vi "Loop_ACT_Claw_Rotation.vi"() -> ()   [LabVIEW 2017, in "Lift.lvlib"]
uses:
  Lift.lvlib
  _SHARE ALL/TypeDef Share All/CLUSTER_TalonInput.ctl
  System Drivers/Phoenix-LabVIEW/Motor Controller/Controls/CTRE_Phoenix_MotorControl_ControlMode.ctl
  _SHARE ALL/RoboRio Share All/SRX Share All/TypeDefs SRX/Cluster_SRX_PIDF.ctl
  _SHARE ALL/TypeDef Share All/CONTROL_PositonGraph.ctl
  CLUSTER_ACT_Lift Output.ctl
  _SHARE ALL/RoboRio Share All/SRX Share All/TypeDefs SRX/Cluster_SRX_General Data.ctl
  _SHARE ALL/RoboRio Share All/SRX Share All/TypeDefs SRX/Cluster_SRX_Common Runtime Data.ctl
  _SHARE ALL/RoboRio Share All/SRX Share All/TypeDefs SRX/Cluster_SRX_Error Calculations.ctl
  _SHARE ALL/RoboRio Share All/SRX Share All/TypeDefs SRX/Cluster_SRX_Voltage Out Data.ctl
  _SHARE ALL/RoboRio Share All/SRX Share All/TypeDefs SRX/Cluster_SRX_Sensor Out Data.ctl
  _SHARE ALL/RoboRio Share All/SRX Share All/TypeDefs SRX/Cluster_SRX_Sensor Quad Data.ctl
  _SHARE ALL/RoboRio Share All/SRX Share All/TypeDefs SRX/Cluster_SRX_Analog In Data.ctl
  _SHARE ALL/RoboRio Share All/SRX Share All/TypeDefs SRX/Cluster_SRX_PWM Sensor Data.ctl
  _SHARE ALL/RoboRio Share All/SRX Share All/TypeDefs SRX/Cluster_SRX_F and R Limit Indicators.ctl
  TypeDef/CLUSTER_PID.ctl
  Globals/Global_Device_IDs.vi
  _SHARE ALL/Global Share All/Global_STOP.vi
  Global_SM Write_Data Out.vi
  Global_ACT Write_Data Out.vi
panel:
  out "Rotation Output":T1 {"Common Runtime Data Out"."Temp" format="%.1f"; "Common Runtime Data Out"."Voltage"."Bus" format="%.3f"; "Common Runtime Data Out"."Voltage"."Output" format="%.3f"; "Common Runtime Data Out"."Voltage"."Percent" format="%.3f"; "Common Runtime Data Out"."Current" format="%.2f"}
  in  "Display Graph":bool
  out "Position Closed Loop Plots":T11
  out "Rotation Input":T12 {"Talon Mode" items=["PercentOutput"=0, "Position"=1, "Velocity"=2, "Current"=3, "Follower"=5, "MotionProfile"=6, "MotionMagic"=7, "MotionMagicArc"=8, "MotionProfileArc"=10, "Disabled"=15]}
  out "Cycle Time (S)":dbl format="%.3g"
  in  "Target Time(ms)":u32=50
  # "C"
  # "Units"
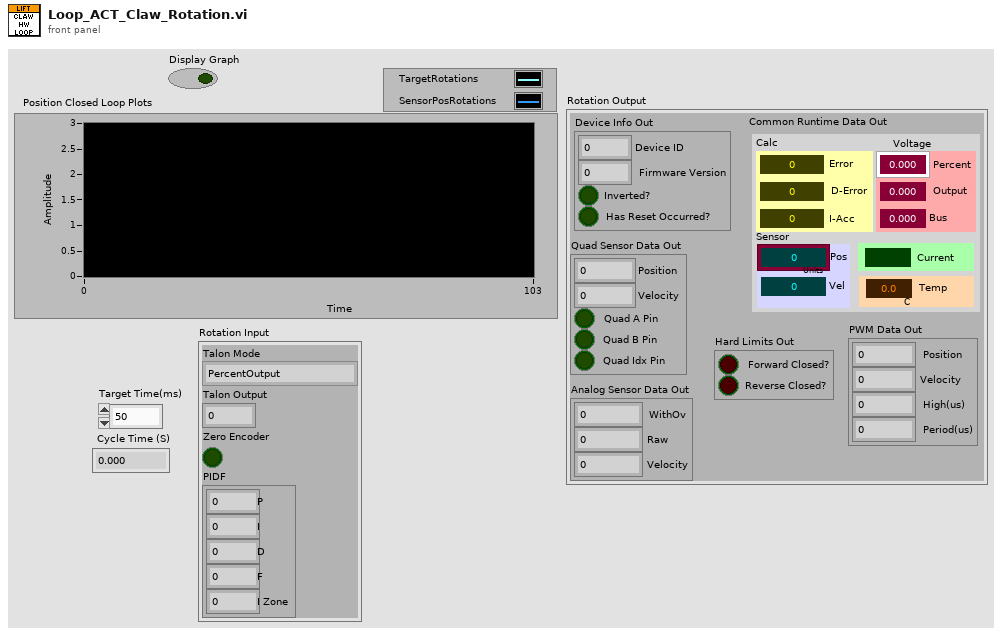
[diagram p1: front panel]
types:
  T1 = typedef "Lift.lvlib/CLUSTER_ACT_Lift Output.ctl" = cluster{"Device Info Out":T2, "Common Runtime Data Out":T3, "Quad Sensor Data Out":T7, "Analog Sensor Data Out":T8, "PWM Data Out":T9, "Hard Limits Out":T10}
  T2 = typedef "Cluster_SRX_General Data.ctl" = cluster{"Device ID":i32, "Firmware Version":i32, "Inverted?":bool, "Has Reset Occurred?":bool}
  T3 = typedef "Cluster_SRX_Common Runtime Data.ctl" = cluster{"Calc":T4, "Voltage ":T5, "Sensor":T6, "Current":dbl, "Temp":dbl}
  T4 = typedef "Cluster_SRX_Error Calculations.ctl" = cluster{"Error":i32, "D-Error":dbl, "I-Acc":dbl}
  T5 = typedef "Cluster_SRX_Voltage Out Data.ctl" = cluster{"Percent":dbl, "Output":dbl, "Bus":dbl}
  T6 = typedef "Cluster_SRX_Sensor Out Data.ctl" = cluster{"Pos":i32, "Vel":i32}
  T7 = typedef "Cluster_SRX_Sensor Quad Data.ctl" = cluster{"Position":i32, "Velocity":i32, "Quad A Pin":bool, "Quad B Pin":bool, "Quad Idx Pin":bool}
  T8 = typedef "Cluster_SRX_Analog In Data.ctl" = cluster{"WithOv":i32, "Raw":i32, "Velocity":i32}
  T9 = typedef "Cluster_SRX_PWM Sensor Data.ctl" = cluster{"Position":i32, "Velocity":i32, "High(us)":i32, "Period(us)":i32}
  T10 = typedef "Cluster_SRX_F and R Limit Indicators.ctl" = cluster{"Forward Closed?":bool, "Reverse Closed?":bool}
  T11 = typedef "CONTROL_PositonGraph.ctl" = cluster{dbl, "Position (Raw Sensor Units)":i32}
  T12 = typedef "CLUSTER_TalonInput.ctl" = cluster{"Talon Mode":T13, "Talon Output":dbl, "Zero Encoder":bool, "PIDF":T14}
  T13 = typedef "CTRE_Phoenix_MotorControl_ControlMode.ctl" = u16
  T14 = typedef "Cluster_SRX_PIDF.ctl" = cluster{"P":dbl, "I":dbl, "D":dbl, "F":dbl, "I Zone":dbl}
  T15 = typedef "CLUSTER_PID.ctl" = cluster{"P":dbl, "I":dbl, "D":dbl, "F":dbl, "I Zone":dbl}
  T16 = typedef "CLUSTER_Arm_Device_IDs.ctl" = cluster{"Rotation Setup":T17, "Telescope Setup":T17, "Rotation Slave Setup":T17, "Telescope Slave Setup":T17, "Claw Rotation Setup":T17}
  T17 = typedef "CLUSTER_Talon_Setup.ctl" = cluster{"Talon SRX ID":u8, "PhaseSensor":bool, "Invert Motor?":bool, "Phoenix Feedback Select":T18, "pidLoopldx":i32, "PID":T15}
  T18 = typedef "CTRE_Phoenix_MotorControl_FeedbackDevice.ctl" = i8
  T19 = typedef "WPI_MotorControlDeviceRef.ctl" = cluster{"DeviceStatus":errorcluster, "Type":T20, "PWM":cluster{"PWM Channel":T21, "DeadBand":T22}, "CAN":cluster{"Device Number":u8, "SetOutput VI Ref":variant, "GetOutput VI Ref":variant, "Enable VI Ref":variant, "Disable VI Ref":variant, "Data":variant}, "Invert":bool, "DIO PWM":cluster{"PWM \"Enable\" Channel":T21, "DIOChannel":T23, "PWM Rate":dbl}}
  T20 = typedef "WPI_MotorControlType.ctl" = enum16{"PWM", "CAN", "DIO PWM"}
  T21 = typedef "FPGA_DIOPWMChannel.ctl" = enum8{"PWM 0", "PWM 1", "PWM 2", "PWM 3", "PWM 4", "PWM 5", "PWM 6", "PWM 7", "PWM 8", "PWM 9", "PWM MXP 0", "PWM MXP 1", "PWM MXP 2", "PWM MXP 3", "PWM MXP 4", "PWM MXP 5", "PWM MXP 6", "PWM MXP 7", "PWM MXP 8", "PWM MXP 9", "Invalid"}
  T22 = typedef "WPI_PWMDeadband.ctl" = cluster{"Name":string, "maxPositivePwm":i32, "minPositivePwm":i32, "centerPwm":i32, "maxNegativePwm":i32, "minNegativePwm":i32, "angularRange":u16}
  T23 = typedef "FPGA_DIOChannel.ctl" = enum8{"DIO 0", "DIO 1", "DIO 2", "DIO 3", "DIO 4", "DIO 5", "DIO 6", "DIO 7", "DIO 8", "DIO 9", "DIO MXP 0", "DIO MXP 1", "DIO MXP 2", "DIO MXP 3", "DIO MXP 4", "DIO MXP 5", "DIO MXP 6", "DIO MXP 7", "DIO MXP 8", "DIO MXP 9", "DIO MXP 10", "DIO MXP 11", "DIO MXP 12", "DIO MXP 13", "DIO MXP 14", "DIO MXP 15", "SPI Port CS1", "SPI Port CS2", "SPI Port CS3", "SPI Port MISO", "SPI Port MOSI", "Invalid"}
  T24 = cluster{"PhoenixMotorControlDevRef":T19, "Claw Rotation Output":T1, "Claw Rotation Input":T12, "Target Time(ms)":u32, "Current Time":timestamp, "Previous Time":timestamp, "Cycle Time (S)":dbl, "Last PID":T15}
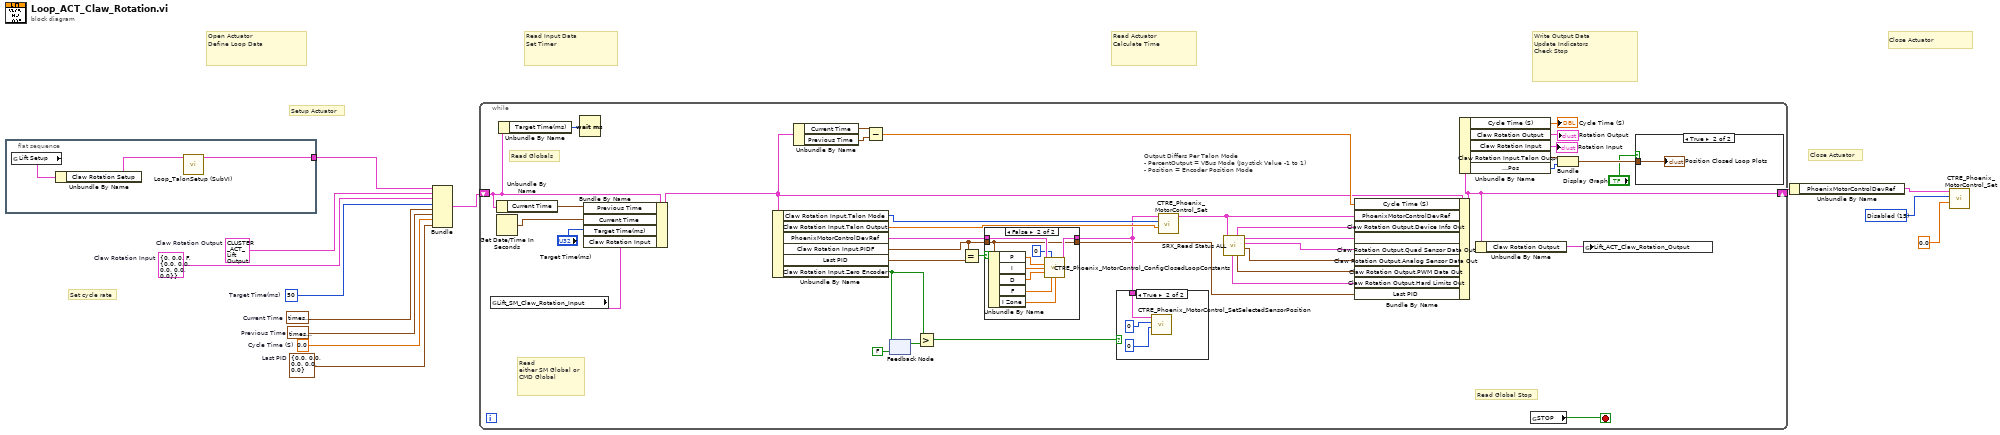
[diagram p0: block diagram]
diagram:
  w1 = T1 {"Device Info Out"={"Device ID"=0, "Firmware Version"=0, "Inverted?"=FALSE, "Has Reset Occurred?"=FALSE}, "Common Runtime Data Out"={"Calc"={"Error"=0, "D-Error"=0.0, "I-Acc"=0.0}, "Voltage "={"Percent"=0.0, "Output"=0.0, "Bus"=0.0}, "Sensor"={"Pos"=0, "Vel"=0}, "Current"=0.0, "Temp"=0.0}, "Quad Sensor Data Out"={"Position"=0, "Velocity"=0, "Quad A Pin"=FALSE, "Quad B Pin"=FALSE, "Quad Idx Pin"=FALSE}, "Analog Sensor Data Out"={"WithOv"=0, "Raw"=0, "Velocity"=0}, "PWM Data Out"={"Position"=0, "Velocity"=0, "High(us)"=0, "Period(us)"=0}, "Hard Limits Out"={"Forward Closed?"=FALSE, "Reverse Closed?"=FALSE}}  # Claw Rotation Output
  w3 = T15 {"P"=0.0, "I"=0.0, "D"=0.0, "F"=0.0, "I Zone"=0.0}  # Last PID
  w5 = T13 15 items=["PercentOutput"=0, "Position"=1, "Velocity"=2, "Current"=3, "Follower"=5, "MotionProfile"=6, "MotionMagic"=7, "MotionMagicArc"=8, "MotionProfileArc"=10, "Disabled"=15] ("Control Mode")
  w7 = T12 {"Talon Mode"=0, "Talon Output"=0.0, "Zero Encoder"=FALSE, "PIDF"={"P"=0.0, "I"=0.0, "D"=0.0, "F"=0.0, "I Zone"=0.0}}  # Claw Rotation Input
  w8 = 0.0  # Cycle Time (S)
  w13 = timestamp(0 s since 1904-01-01)  # Previous Time
  w12 = timestamp(0 s since 1904-01-01)  # Current Time
  w11 = u32 50  # Target Time(ms)
  # "Close Actuator"
  # "Write Output Data\nUpdate Indicators\nCheck Stop"
  # "Read Actuator\nCalculate Time"
  # "Read Input Data\nSet Timer"
  # "Open Actuator\nDefine Loop Data"
  # "Set cycle rate"
  # "Close Actuator"
  # "Setup Actuator"
  n1 = flat-sequence {
    tunnel: [w14] -> w2
    frame #0 {
      n2 = global read "Global_Device_IDs.vi" "Lift Setup"() -> (w16:T16)
      n3 = Unbundle By Name(w16) -> ("Claw Rotation Setup"=w15:T17)
      n4 = call "Loop_TalonSetup (SubVI).vi"("Talon Setup"=w15) -> ("PhoenixMotorControlDevRef"=w14:T19)  [unwired: 10 in]
    }
  }
  n5 = Bundle("PhoenixMotorControlDevRef"=w2, "Claw Rotation Output"=w1, "Claw Rotation Input"=w7, "Target Time(ms)"=w11, "Current Time"=w12, "Previous Time"=w13, "Cycle Time (S)"=w8, "Last PID"=w3) -> (w10:T24)  [unwired: 1 in]
  n6 = while {
    shift-right: [w47] -> w9
    shift-left: w10 -> [w49]
    stop <- w55 stop-if-true
    # "Output Differs Per Talon Mode\n- PercentOutput = VBus Mode (Joystick Value -1 to 1)\n- Position = Encoder Position Mode"
    # "Read\neither SM Global or CMD Global"
    # "Read Globals"
    # "Read Global Stop"
    n7 = global read "Global_SM Write_Data Out.vi" "Lift_SM_Claw_Rotation_Input"() -> (w43:T12)
    n8 = Unbundle By Name(w49) -> ("Current Time"=w53:timestamp)
    n9 = Get Date/Time In Seconds() -> (seconds since 1Jan1904=w54:timestamp)
    n10 = Unbundle By Name(w49) -> ("Target Time(ms)"=w48:u32)
    n11 = Wait (ms)(milliseconds to wait=w48) -> ()  [unwired: 1 out]
    n12 = Bundle By Name(cluster=w49, "Previous Time"=w53, "Current Time"=w54, "Target Time(ms)"="Target Time(ms)", "Claw Rotation Input"=w43) -> (w36:T24)
    n13 = Unbundle By Name(w36) -> ("Claw Rotation Input.Talon Mode"=w42:T13, "Claw Rotation Input.Talon Output"=w41:dbl, "PhoenixMotorControlDevRef"=w35:T19, "Claw Rotation Input.PIDF"=w31:T14, "Last PID"=w32:T15, "Claw Rotation Input.Zero Encoder"=w27:bool)
    n14 = Unbundle By Name(w36) -> ("Current Time"=w52:timestamp, "Previous Time"=w51:timestamp)
    n15 = Subtract(x=w52, y=w51) -> (x-y=w45:dbl)
    n16 = feedback #1(FALSE) -> (w28:bool)
    n17 = feedback-in #1(w27) -> ()
    n18 = Greater?(x=w27, y=w28) -> (0:w26:bool)
    n19 = Equal?(x=w31, y=w32) -> (x = y?=w30:bool)
    n20 = case shown="False" w30 {
      tunnel: w35 -> [w57 w66]
      tunnel: [w57 w65] -> w34
      tunnel: w31 -> [w56 w58]
      tunnel: [w56 w58] -> w18
      frame True {
      }
      frame False {
        n21 = Unbundle By Name(w58) -> ("P"=w63:dbl, "I"=w62:dbl, "D"=w61:dbl, "F"=w60:dbl, "I Zone"=w59:dbl)
        n22 = call "CTRE_Phoenix_MotorControl_ConfigClosedLoopConstants.vi"("PhoenixMotorControlDevRef"=w66, "slotIdx"=0, "P"=w63, "I"=w62, "D"=w61, "F"=w60, "I Zone"=w59) -> ("PhoenixMotorControlDevRef"=w65:T19)  [unwired: 7 in, 1 out]
      }
    }
    n23 = case shown="True" w26 {
      tunnel: w34 -> [_ w70]
      frame False {
      }
      frame True {
        n24 = call "CTRE_Phoenix_MotorControl_SetSelectedSensorPosition.vi"("pidLoopIdx"=u32 0, "New Sensor Position"=0, "PhoenixMotorControlDevRef"=w70) -> ()  [unwired: 7 in, 2 out]
      }
    }
    n25 = call "CTRE_Phoenix_MotorControl_Set.vi"("Output"=w41, "Control Mode"=w42, "PhoenixMotorControlDevRef"=w34) -> ("PhoenixMotorControlDevRef"=w25:T19)  [unwired: 7 in, 1 out]
    n26 = call "SRX_Read Status ALL.vi"("PhoenixMotorControlDevRef"=w25) -> ("Analog Sensor Data Out"=w21:T8, "Quad Sensor Data Out"=w22:T7, "Common Runtime Data Out"=w23:T3, "PWM Data Out"=w20:T9, "Device Info Out"=w24:T2, "Hard Limits Out"=w19:T10)  [unwired: 4 in, 1 out]
    n27 = Bundle By Name(cluster=w36, "Cycle Time (S)"=w45, "PhoenixMotorControlDevRef"=w25, "Claw Rotation Output.Device Info Out"=w24, "Claw Rotation Output.Common Runtime Data Out"=w23, "Claw Rotation Output.Quad Sensor Data Out"=w22, "Claw Rotation Output.Analog Sensor Data Out"=w21, "Claw Rotation Output.PWM Data Out"=w20, "Claw Rotation Output.Hard Limits Out"=w19, "Last PID"=w18) -> (w47:T24)
    n28 = Unbundle By Name(w47) -> ("Cycle Time (S)"=→"Cycle Time (S)":dbl, "Claw Rotation Output"=→"Rotation Output":T1, "Claw Rotation Input"=→"Rotation Input":T12, "Claw Rotation Input.Talon Output"=w39:dbl, "Claw Rotation Output.Common Runtime Data Out.Sensor.Pos"=w38:i32)
    n29 = Unbundle By Name(w47) -> ("Claw Rotation Output"=w44:T1)
    n30 = global read "Global_STOP.vi" "STOP"() -> (w55:bool)
    n31 = Bundle("Talon Output"=w39, "Pos"=w38) -> (w37:cluster{"Talon Output":dbl, "Pos":i32})  [unwired: 1 in]
    n32 = global write "Global_ACT Write_Data Out.vi" "Lift_ACT_Claw_Rotation_Output"(w44) -> ()
    n33 = case shown="True" "Display Graph" {
      tunnel: w37 -> [_ w67]
      frame False {
      }
      frame True {
        "Position Closed Loop Plots" <- w67
      }
    }
  }
  n34 = Unbundle By Name(w9) -> ("PhoenixMotorControlDevRef"=w6:T19)
  n35 = call "CTRE_Phoenix_MotorControl_Set.vi"("Output"=0.0, "Control Mode"=w5, "PhoenixMotorControlDevRef"=w6) -> ()  [unwired: 7 in, 2 out]
